vi "lvgit pull.vi"(8 "error in":errorcluster, 11 "path":path) -> (0 "error out":errorcluster)   [LabVIEW 2017]
uses:
  <vilib>/Hampel Software Engineering/Git API/Git API/GIT-api.lvclass/GIT-api.ctl
  <vilib>/Hampel Software Engineering/Git API/Git API/Accessors/GIT-Set Working Dir.vi
  <vilib>/Hampel Software Engineering/Git API/Git API/GIT-api.lvclass
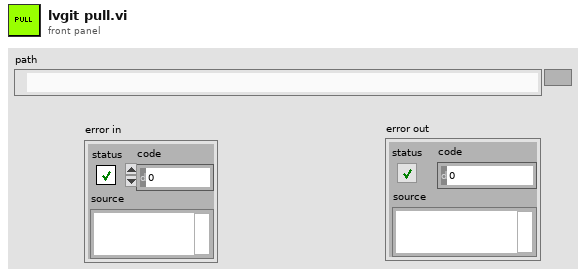
[diagram p1: front panel]
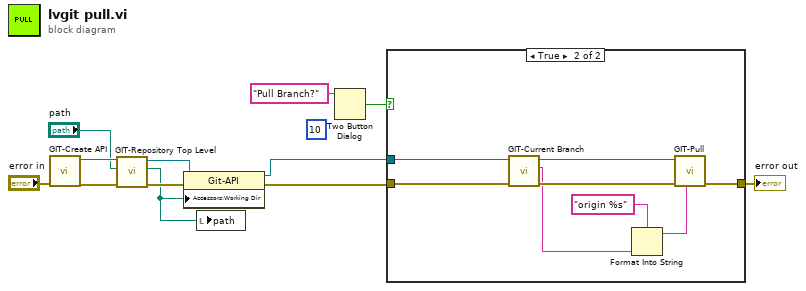
[diagram p0: block diagram]
diagram:
  (unwired) 10 ("F Timeout(-1 s)")
  n1 = call <vilib>:"GIT-Create API.vi"("error in"="error in") -> ("error out"=w9:errorcluster, "git-api out"=w10:refnum<class "GIT-api.lvclass">)  [unwired: 9 in]
  n2 = call <vilib>:"GIT-Repository Top Level.vi"("error in"=w9, "Current Path"="path", "git-api in"=w10) -> ("error out"=w12:errorcluster, "Repo Top Level Path"=w3:path, "git-api out"=w11:refnum<class "GIT-api.lvclass">)  [unwired: 6 in]
  n3 = property class="Git-API"(reference=w11, error in=w12, "Accessors:Working Dir"=w3) -> (reference out=w7:refnum<class "GIT-api.lvclass">, error out=w8:errorcluster)
  n4 = local write "path"(w3) -> ()
  n5 = Two Button Dialog(message="Pull Branch?") -> (T button?=w4:bool)  [unwired: 2 in]
  n6 = case shown="True" w4 {
    tunnel: w8 -> [w13 w19]
    tunnel: [w13 w21] -> w1
    tunnel: w7 -> [_ w20]
    frame False {
    }
    frame True {
      n7 = call <vilib>:"GIT-Current Branch.vi"("error in"=w19, "git-api in"=w20) -> ("error out"=w17:errorcluster, "current branch"=w14:string, "git-api out"=w18:refnum<class "GIT-api.lvclass">)  [unwired: 7 in]
      n8 = Format Into String(format string="origin %s" ("param"), w14) -> (resulting string=w15:string)  [unwired: 2 in, 1 out]
      n9 = call <vilib>:"GIT-Pull.vi"("param"=w15, "error in"=w17, "git-api in"=w18) -> ("error out"=w21:errorcluster)  [unwired: 7 in, 1 out]
    }
  }
  "error out" <- w1
